vi "Process Lidar Data.vi"(6 "Estimated Pose After Scan":cluster{"X":dbl, "Y":dbl, "R":dbl}, 7 "Estimated Pose Before Scan":cluster{"X":dbl, "Y":dbl, "R":dbl}, 8 "Lidar Offset from Center of Rotation (mm)":dbl=-100.0 format="%#_13g", 9 "Direction":dbl[](array[numeric]), 10 "Magnitude":dbl[](array[numeric]), 11 "path in":path) -> (2 "Data Comparison":cluster{"X":dbl[], "Y":dbl[]}[](array[cluster]), 3 "Lidar Scan":T1)   [LabVIEW 2017]
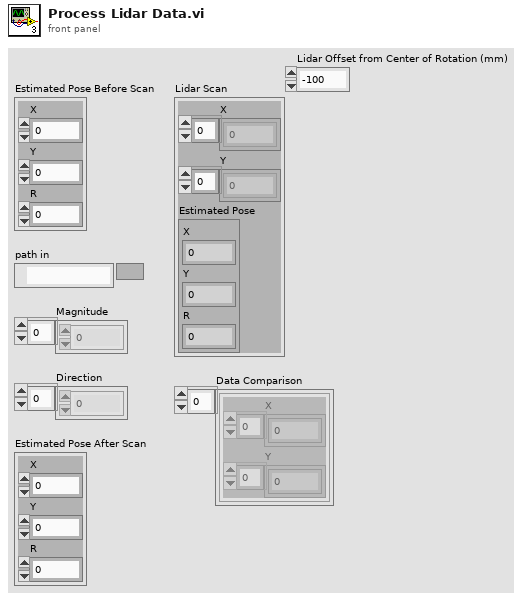
[diagram p1: front panel]
types:
  T1 = cluster{"X":dbl[], "Y":dbl[], "Estimated Pose":cluster{"X":dbl, "Y":dbl, "R":dbl}}
  T2 = cluster{"X":dbl[], "Y":dbl[], "Estimated Pose After Scan":cluster{"X":dbl, "Y":dbl, "R":dbl}}
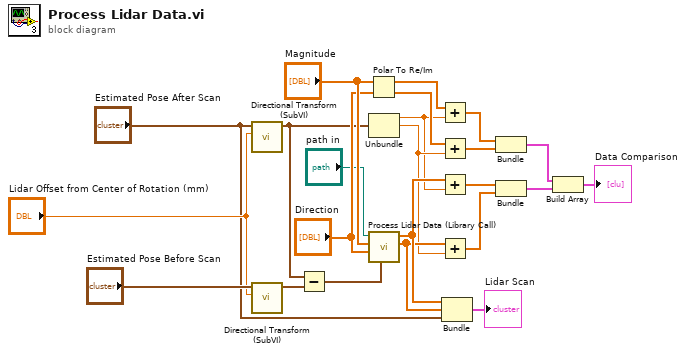
[diagram p0: block diagram]
diagram:
  n1 = call "Directional Transform (SubVI).vi"("Transform Amount (mm)"="Lidar Offset from Center of Rotation (mm)", "Pose"="Estimated Pose After Scan") -> ("Pose"=w1:cluster{"X":dbl, "Y":dbl, "R":dbl})  [unwired: 9 in]
  n2 = call "Directional Transform (SubVI).vi"("Transform Amount (mm)"="Lidar Offset from Center of Rotation (mm)", "Pose"="Estimated Pose Before Scan") -> ("Pose"=w16:cluster{"X":dbl, "Y":dbl, "R":dbl})  [unwired: 9 in]
  n3 = Subtract(x=w1, y=w16) -> (x-y=w18:cluster{"X":dbl, "Y":dbl, "R":dbl})
  n4 = Polar To Re/Im(2:"Direction", 3:"Magnitude") -> (0:w8:dbl[], 1:w11:dbl[])
  n5 = Unbundle(w1) -> ("X"=w4:dbl, "Y"=w5:dbl)  [unwired: 1 out]
  n6 = call "Process Lidar Data (Library Call).vi"("Pose Delta"=w18, "Direction"="Direction", "Magnitude"="Magnitude", "Library Path"="path in") -> ("Y"=w6:dbl[], "X"=w7:dbl[])  [unwired: 6 in]
  n7 = Add(x=w11, y=w4) -> (x+y=w10:dbl[])
  n8 = Add(x=w8, y=w5) -> (x+y=w9:dbl[])
  n9 = Add(x=w7, y=w4) -> (x+y=w3:dbl[])
  n10 = Add(x=w6, y=w5) -> (x+y=w2:dbl[])
  n11 = Bundle("X"=w7, "Y"=w6, "Estimated Pose After Scan"="Estimated Pose After Scan") -> (→"Lidar Scan":T2)  [unwired: 1 in]
  n12 = Bundle(w10, w9) -> (w13:cluster{dbl[], dbl[]})  [unwired: 1 in]
  n13 = Bundle(w3, w2) -> (w12:cluster{dbl[], dbl[]})  [unwired: 1 in]
  n14 = Build Array(w13, w12) -> (→"Data Comparison":cluster{dbl[], dbl[]}[])
